vi "reset_TRIG1.vi"(8 "error in (no error)":errorcluster, 11 "VISA resource name":refnum<visa-resource-name>) -> (0 "error out":errorcluster, 3 "VISA resource name out":refnum<visa-resource-name>)   [LabVIEW 2012]
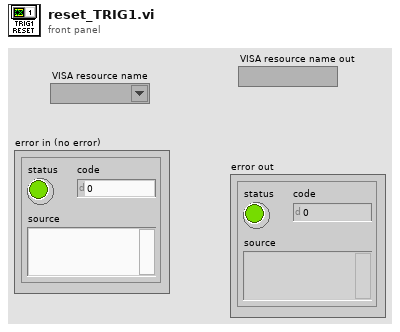
[diagram p1: front panel]
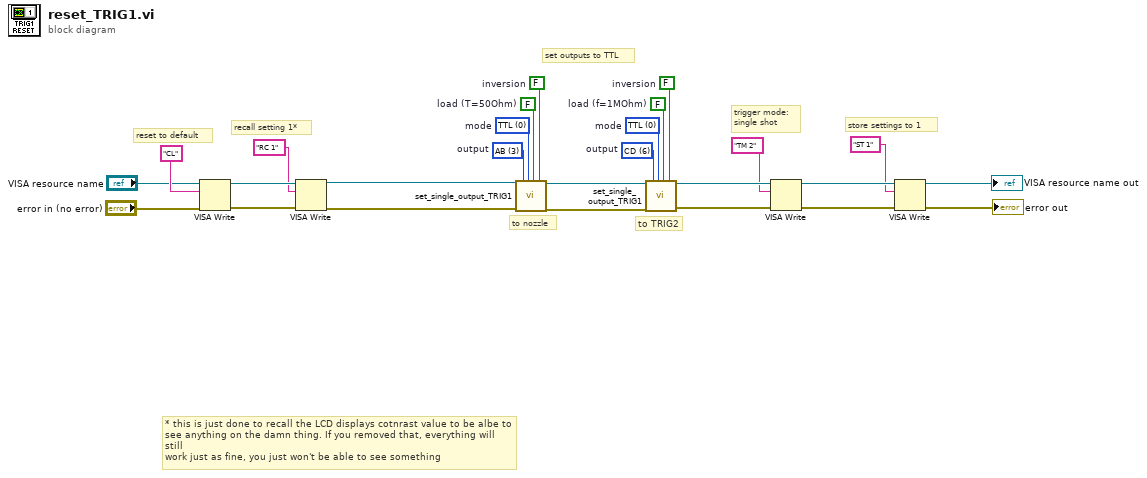
[diagram p0: block diagram]
diagram:
  w15 = FALSE  # inversion
  w16 = FALSE  # load (f=1MOhm)
  w17 = 0 items=["TTL", "NIM", "ECL", "VAR"]  # mode
  w18 = u16 6 items=["T0", "A", "B", "AB", "C", "D", "CD"]  # output
  w19 = FALSE  # inversion
  w20 = FALSE  # load (T=50Ohm)
  w21 = 0 items=["TTL", "NIM", "ECL", "VAR"]  # mode
  w22 = u16 3 items=["T0", "A", "B", "AB", "C", "D", "CD"]  # output
  # "store settings to 1"
  # "trigger mode:\nsingle shot"
  # "to TRIG2"
  # "to nozzle"
  # "set outputs to TTL"
  # "* this is just done to recall the LCD displays cotnrast value to be albe to \nsee anything on the damn thing. If you removed that, everything will still\nwork just as fine, you just won't be able to see something"
  # "recall setting 1*"
  # "reset to default"
  n1 = VISA Write(VISA resource name="VISA resource name", write buffer="CL", error in (no error)="error in (no error)") -> (VISA resource name out=w25:refnum<visa-resource-name>, error out=w24:errorcluster)  [unwired: 1 out]
  n2 = VISA Write(VISA resource name=w25, write buffer="RC 1", error in (no error)=w24) -> (VISA resource name out=w1:refnum<visa-resource-name>, error out=w2:errorcluster)  [unwired: 1 out]
  n3 = call "set_single_output_TRIG1.vi"("VISA resource name"=w1, "error in"=w2, "output"=w22, "mode"=w21, "load"=w20, "inversion"=w19) -> ("VISA resource out"=w14:refnum<visa-resource-name>, "error out"=w12:errorcluster)  [unwired: 12 in]
  n4 = call "set_single_output_TRIG1.vi"("VISA resource name"=w14, "error in"=w12, "output"=w18, "mode"=w17, "load"=w16, "inversion"=w15) -> ("VISA resource out"=w10:refnum<visa-resource-name>, "error out"=w13:errorcluster)  [unwired: 12 in]
  n5 = VISA Write(VISA resource name=w10, write buffer="TM 2", error in (no error)=w13) -> (VISA resource name out=w7:refnum<visa-resource-name>, error out=w11:errorcluster)  [unwired: 1 out]
  n6 = VISA Write(VISA resource name=w7, write buffer="ST 1", error in (no error)=w11) -> (VISA resource name out=→"VISA resource name out":refnum<visa-resource-name>, error out=→"error out":errorcluster)  [unwired: 1 out]
